vi "set enter.vi"(8 "error in":errorcluster, 10 "nextstate in":T1=enum."Withdraw", 11 "enterstate":T2) -> (0 "error out":errorcluster, 3 "nextstate out":T1=enum."Withdraw")   [LabVIEW 2015]
doc: "Remember naext action. After action when necessary is pressing Enter after pressing another button."
uses:
  controls/enterstatus.ctl
  controls/nextstate.ctl
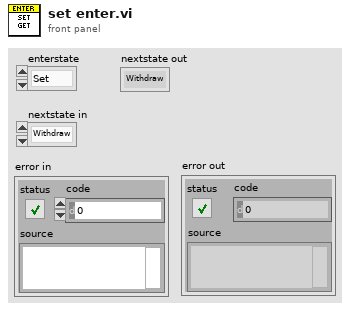
[diagram p1: front panel]
types:
  T1 = typedef "nextstate.ctl" = enum16{"Fast Cash", "Withdraw", "Deposit", "Validate"}
  T2 = typedef "enterstatus.ctl" = enum16{"Set", "Get"}
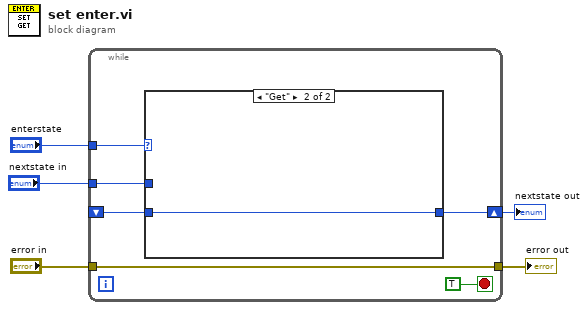
[diagram p0: block diagram]
diagram:
  n1 = while {
    tunnel: "enterstate" -> [w10]
    shift-right: [w8] -> w5
    shift-left: _ -> [w9]
    tunnel: "nextstate in" -> [w7]
    tunnel: [w6] -> w1
    tunnel: "error in" -> [w6]
    stop <- TRUE stop-if-true
    n2 = case shown="\"Get\"" w10 {
      tunnel: w9 -> [_ w13]
      tunnel: [w12 w13] -> w8
      tunnel: w7 -> [w12 _]
      frame "Set", Default {
      }
      frame "Get" {
      }
    }
  }
  "nextstate out" <- w5
  "error out" <- w1
